vi "DHE_DO_IMREAD_NORMAL.vi"(8 "error in":errorcluster) -> (0 "error out":errorcluster, 2 "response":string)   [LabVIEW 2016]
uses:
  Common/public/vis/CMN_FVAR_action.ctl
  SDSU_GBLVariables.vi
  DBSHAND/private/vis/DatabaseHand_Element_Get(bool).vi
  DBSHAND/private/vis/DatabaseHand_Element_Get(double).vi
  DBSHAND/private/vis/DatabaseHand_Element_Set(double).vi
  c/lib/libarcDHE.so
panel:
  out "error out 2":errorcluster
  out "remaining elements":string[](array[string])
  in  "stop":bool
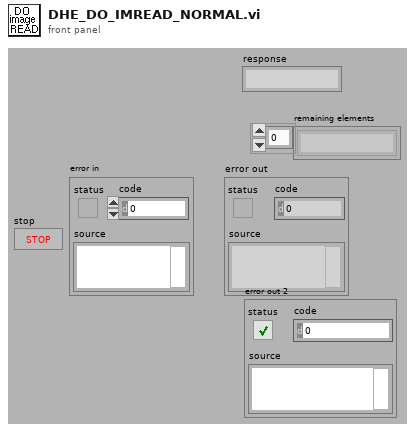
[diagram p1: front panel]
types:
  T1 = typedef "DatabaseHand_RefNum.ctl" = refnum<vi>
  T2 = enum16{"Idle", "Exposing", "Paused", "AbortExp", "Reading", "AbortRead", "FinishedReading", "Resetting", "Reducing"}
  T3 = cluster{"Video Processor Type":string, "support gain":bool, "Timing Board":string, "support reset":bool, "Utility Board":string, "Shutter":string, "Temperature":string, "support temp control":bool, "Detector Type":string, "Support MPP":string, "Support Binning":string, "Readout Mode":string, "support shutter control":bool}
  T4 = typedef "CMN_Buffers.ctl" = cluster{"TotalPixels":u32, "Total image bytes":u32, "Total Phys Buffers":u32, "virtual buf pixels":u32, "virtual bytes size":u32, "Remaining piece":u32, "Transfer_Buf_size":u32}
  T5 = typedef "CMN_TimingInfo.ctl" = cluster{"PixelTime":sgl, "SkipPixel":sgl, "SkipRow":sgl, "ShiftRow":sgl, "ShiftedPix":u16, "known_overhead":sgl, "DET_READ_TIME":sgl}
  T6 = typedef "CMN_FVAR_action.ctl" = enum16{"read", "write"}
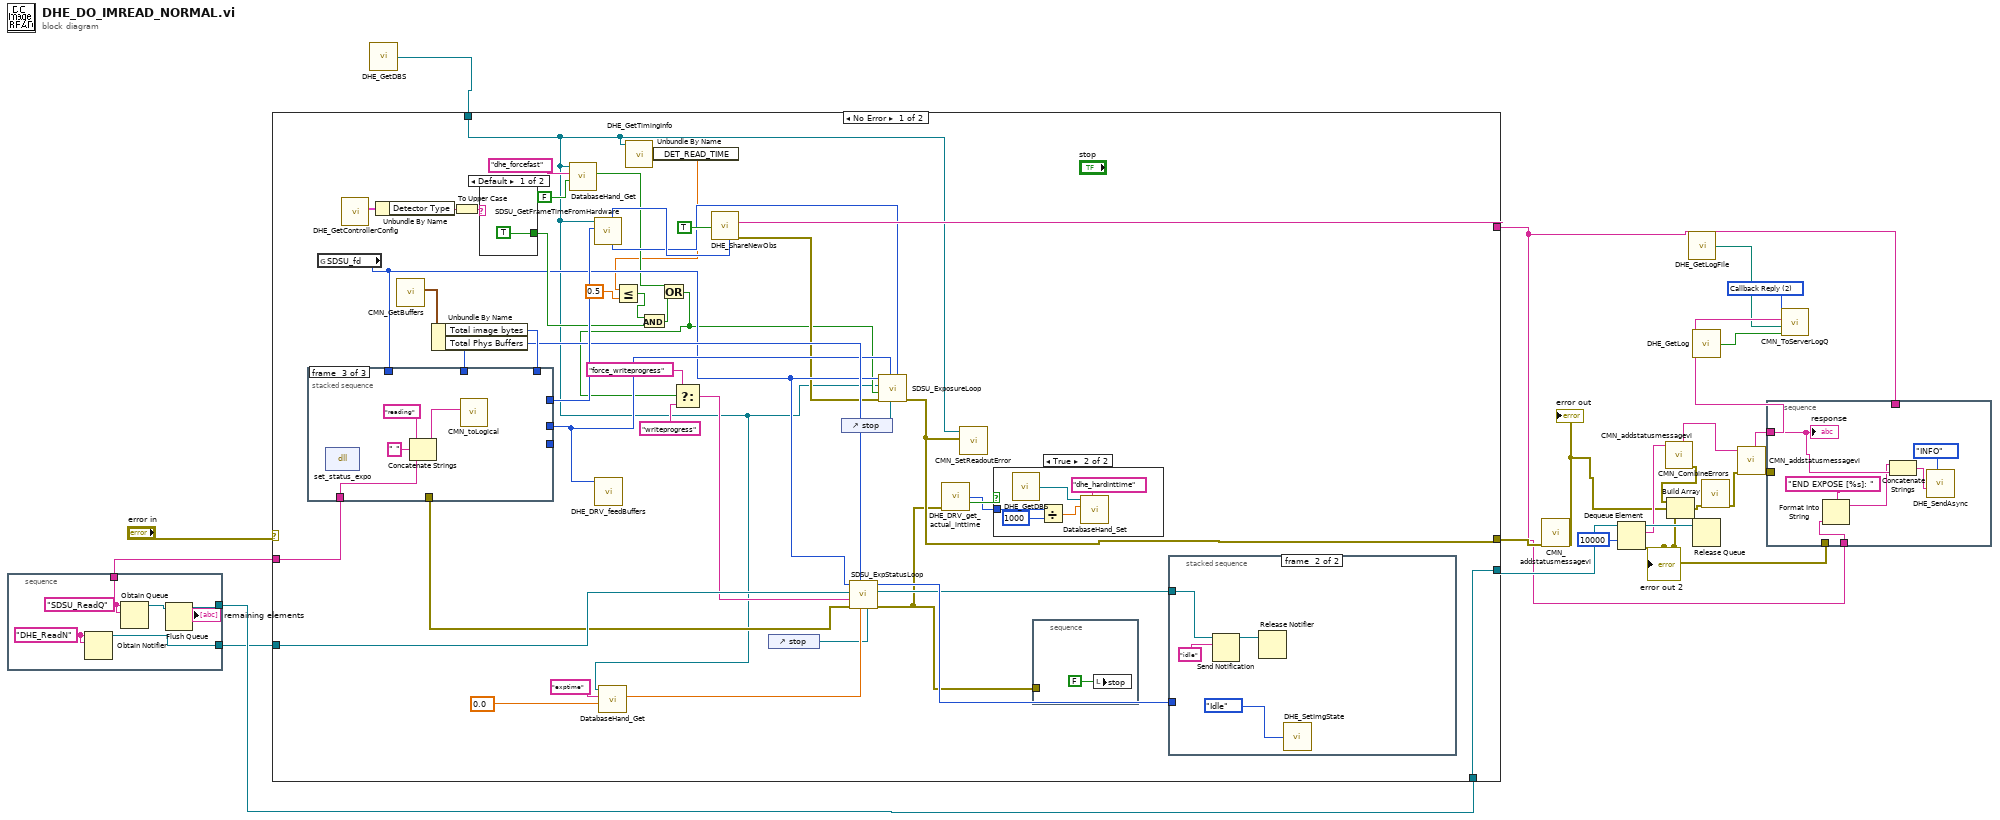
[diagram p0: block diagram]
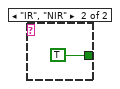
[diagram p3: hidden frame]
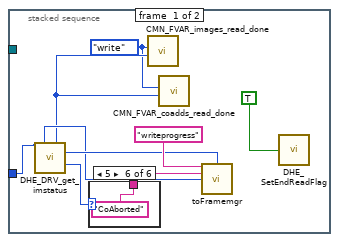
[diagram p4: hidden frame]
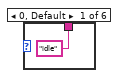
[diagram p5: hidden frame]
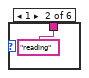
[diagram p6: hidden frame]
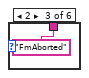
[diagram p7: hidden frame]
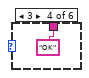
[diagram p8: hidden frame]
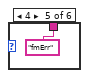
[diagram p9: hidden frame]
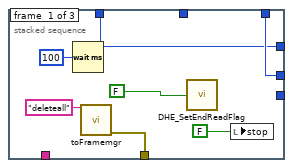
[diagram p10: hidden frame]
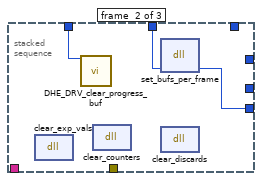
[diagram p11: hidden frame]
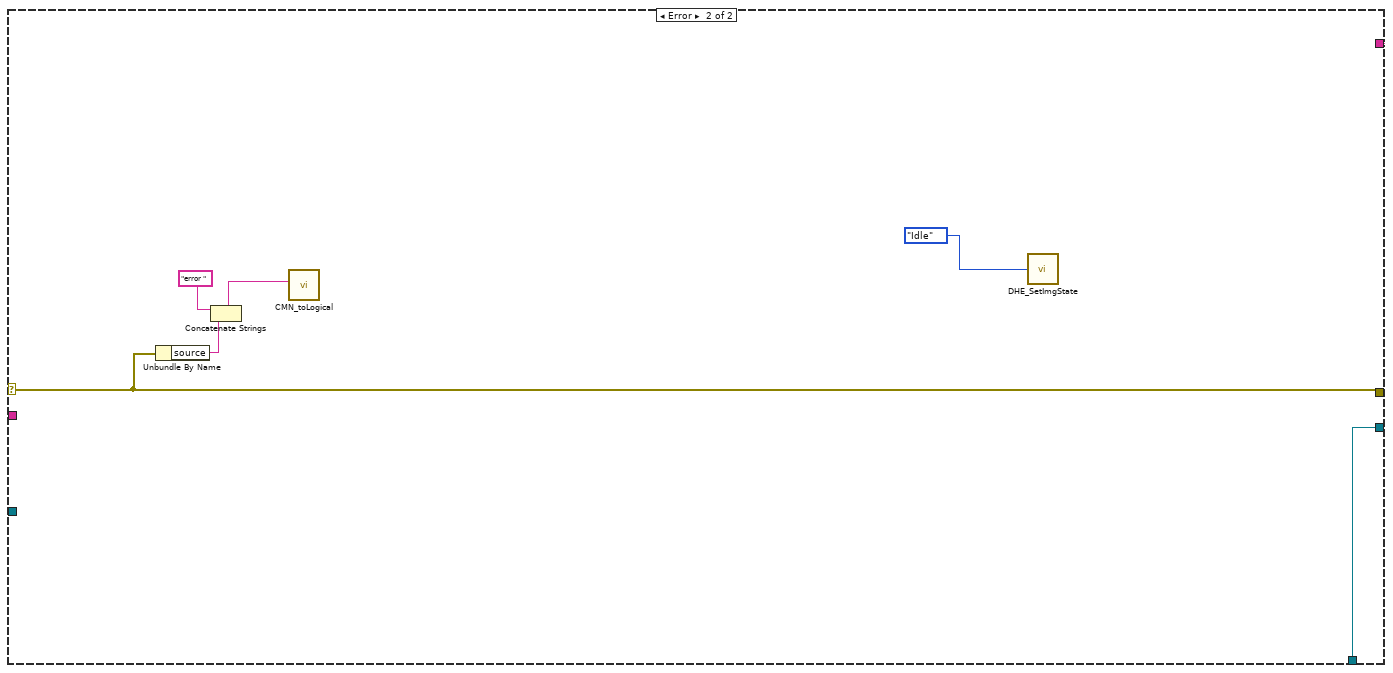
[diagram p12: hidden frame]
diagram:
  w19 = u16 2 items=["command", "imediateReply", "Callback Reply", "Information"] ("type")
  n1 = stacked-sequence {
    tunnel: [w28] -> w20
    tunnel: [w26] -> w15
    tunnel: [w23] -> w8
    frame #0 {
      w24 = "DHE_ReadN" ("name (unnamed)")
      w28 = "SDSU_ReadQ" ("name (unnamed)")
      n2 = Obtain Notifier(name (unnamed)=w24, notification data type=w24) -> (notifier out=w23:refnum<notifier>)  [unwired: 2 in, 2 out]
      n3 = Obtain Queue(name (unnamed)=w28, element data type=w28) -> (queue out=w27:refnum<queue>)  [unwired: 3 in, 2 out]
      n4 = Flush Queue(queue=w27) -> (queue out=w26:refnum<queue>, remaining elements=→"remaining elements":string[])  [unwired: 1 in, 1 out]
    }
  }
  n5 = call "DHE_GetDBS.vi"() -> ("DHE_DBSRef"=w5:T1)  [unwired: 9 out]
  n6 = case shown="No Error" "error in" {
    selector: "error in" -> [_ w118]
    tunnel: [w47 w118] -> w18
    tunnel: w5 -> [w34 _]
    tunnel: w20 -> [w68 _]
    tunnel: [w67 w115] -> w14
    tunnel: w15 -> [w67 w115]
    tunnel: w8 -> [w54 _]
    tunnel: [w62 "" ("obsID")] -> w2
    frame No Error {
      n7 = global read "SDSU_GBLVariables.vi" "SDSU_fd"() -> (w44:i32)
      n8 = call "DHE_GetControllerConfig.vi"() -> ("ControllerConfigCluster"=w58:T3)  [unwired: 11 out]
      n9 = Unbundle By Name(w58) -> ("Detector Type"=w57:string)
      n10 = call "CMN_GetBuffers.vi"() -> ("BuffersDimensions"=w69:T4)  [unwired: 2 in, 9 out]
      n11 = Unbundle By Name(w69) -> ("Total image bytes"=w66:u32, "Total Phys Buffers"=w52:u32)
      n12 = stacked-sequence {
        tunnel: [_ w106 _] -> _
        tunnel: w52 -> [_ w108 _]
        tunnel: w44 -> [w102 w107 _]
        tunnel: w68 -> [_ _ w110]
        tunnel: [w104 _ _] -> w45
        tunnel: w66 -> [w104 _ _]
        tunnel: [w102 _ _] -> w65
        tunnel: [w99 _ _] -> w48
        frame #0 {
          n13 = Wait (ms)(milliseconds to wait=u32 100) -> ()  [unwired: 1 out]
          n14 = call "toFramemgr.vi"("command"="deleteall") -> ("error out"=w99:errorcluster)  [unwired: 8 in, 6 out]
          n15 = call "DHE_SetEndReadFlag.vi"("DHE_read_ended"=FALSE ("readout ended")) -> ()  [unwired: 9 out]
          n16 = local write "stop"(FALSE ("stop")) -> ()
        }
        frame #1 {
          n17 = dll-call lib="home/simager/panview/PAN/Modules/SDSU/private/c/lib/libarcDHE.so" fn="clear_exp_vals"() -> ()  [unwired: 3 in, 3 out]
          n18 = call "DHE_DRV_clear_progress_buf.vi"("fd"=w107) -> ()  [unwired: 1 in, 14 out]
          n19 = dll-call lib="home/simager/panview/PAN/Modules/SDSU/private/c/lib/libarcDHE.so" fn="clear_counters"() -> ()  [unwired: 3 in, 3 out]
          n20 = dll-call lib="home/simager/panview/PAN/Modules/SDSU/private/c/lib/libarcDHE.so" fn="set_bufs_per_frame" label="bufs_per_frame"("total_bufs"=w108) -> ("total_bufs"=w106:i32)  [unwired: 3 in, 3 out]
          n21 = dll-call lib="home/simager/panview/PAN/Modules/SDSU/private/c/lib/libarcDHE.so" fn="clear_discards"() -> ()  [unwired: 3 in, 3 out]
        }
        frame #2 {
          n22 = dll-call lib="home/simager/panview/PAN/Modules/SDSU/private/c/lib/libarcDHE.so" fn="set_status_expo"() -> ()  [unwired: 3 in, 3 out]
          n23 = Concatenate Strings("reading" ("command"), " " ("string"), w110) -> (w109:string)
          n24 = call "CMN_toLogical.vi"("command"=w109) -> ()  [unwired: 10 out]
        }
      }
      n25 = To Upper Case(1:w57) -> (0:w56:string)
      n26 = case shown="Default" w56 {
        tunnel: [TRUE TRUE] -> w55
        frame Default {
        }
        frame "IR", "NIR" {
        }
      }
      n27 = call-poly "DatabaseHand_Get.vi"("default value"=FALSE ("async?"), "name"="dhe_forcefast", "Database RefNum in"=w34) -> ("value"=w36:bool)  [unwired: 2 in, 6 out]
      n28 = call "SDSU_GetFrameTimeFromHardware.vi"("fd"=w65, "Database Ref"=w34) -> ("idle time"=w43:u32, "total exp time"=w64:u32)  [unwired: 1 in, 7 out]
      n29 = call "DHE_DRV_feedBuffers.vi"("bufsize"=w45) -> ()  [unwired: 10 out]
      n30 = call-poly "DatabaseHand_Get.vi"("default value"=0.0, "name"="exptime", "Database RefNum in"=w34) -> ("value"=w51:dbl)  [unwired: 2 in, 6 out]
      n31 = call "DHE_GetTimingInfo.vi"("Database RefNum out"=w34) -> ("Timing"=w33:T5)  [unwired: 10 out]
      n32 = Unbundle By Name(w33) -> ("DET_READ_TIME"=w32:sgl)
      n33 = Less Or Equal?(x=w32, y=0.5) -> (x <= y?=w39:bool)
      n34 = And(x=w39, y=w55) -> (x .and. y?=w38:bool)
      n35 = Or(x=w36, y=w38) -> (x .or. y?=w37:bool)
      n36 = Select(t="force_writeprogress" ("command"), s=w37, f="writeprogress" ("command")) -> (s? t:f=w53:string)
      n37 = call "DHE_ShareNewObs.vi"("exptime (ms)"=w64, "async?"=TRUE) -> ("error out"=w42:errorcluster, "obsID"=w62:string)  [unwired: 1 in, 7 out]
      n38 = control-ref of="stop"() -> (w50:refnum<vi>)
      n39 = control-ref of="stop"() -> (w46:refnum<vi>)
      n40 = call "SDSU_ExpStatusLoop.vi"("stop ref"=w50, "exptime"=w51, "Total Phys Buffers"=w52, "error in (no error)"=w48, "frames command"=w53, "notifier"=w54, "fd"=w44) -> ("error out"=w29:errorcluster, "notifier  out"=w35:refnum<notifier>, "fd out"=w49:i32)  [unwired: 2 out]
      n41 = call "SDSU_ExposureLoop.vi"("idle time"=w43, "stop ref"=w46, "Total image bytes"=w45, "error IO"=w42, "fast"=w37, "Database RefNum in"=w34, "SDSU_fd"=w44) -> ("error out"=w47:errorcluster)  [unwired: 4 out]
      n42 = call "DHE_DRV_get_actual_inttime.vi"("error in (no error)"=w29) -> ("actual inttime"=w30:i32, "supported"=w31:bool)  [unwired: 13 out]
      n43 = call "CMN_SetReadoutError.vi"("readout error"=w47, "Database RefNum in"=w34) -> ()  [unwired: 1 in, 9 out]
      n44 = case shown="True" w31 {
        tunnel: w30 -> [_ w74]
        frame False {
        }
        frame True {
          n45 = call "DHE_GetDBS.vi"() -> ("DHE_DBSRef"=w76:T1)  [unwired: 9 out]
          n46 = Divide(x=w74, y=1000) -> (x/y=w72:dbl)
          n47 = call-poly "DatabaseHand_Set.vi"("name"="dhe_hardinttime", "value"=w72, "Database RefNum in"=w76) -> ()  [unwired: 5 in, 4 out]
        }
      }
      n48 = stacked-sequence {
        tunnel: w29 -> [_]
        frame #0 {
          n49 = local write "stop"(FALSE ("stop")) -> ()
        }
      }
      n50 = stacked-sequence {
        tunnel: w49 -> [w87 _]
        tunnel: w35 -> [_ w95]
        frame #0 {
          w80 = CMN_FVAR_action."write" ("action")
          n51 = call "DHE_DRV_get_imstatus.vi"("fd"=w87) -> ("ptr to buffer"=w83:u64, "buff read"=w84:i32, "frame status"=w86:i32, "images done"=w81:i32)  [unwired: 1 in, 10 out]
          n52 = case shown="5" w86 {
            tunnel: ["idle" "reading" "FmAborted" "OK" "fmErr" "CoAborted"] -> w85
            frame 0, Default {
            }
            frame 1 {
            }
            frame 2 {
            }
            frame 3 {
            }
            frame 4 {
            }
            frame 5 {
            }
          }
          n53 = call "CMN_FVAR_images_read_done.vi"("value in"=w81, "action"=w80) -> ()  [unwired: 9 out]
          n54 = call "CMN_FVAR_coadds_read_done.vi"("value in"=w81, "action"=w80) -> ()  [unwired: 9 out]
          n55 = call "toFramemgr.vi"("command"="writeprogress", "progress"=w84, "arg"=w85, "bufpointer"=w83) -> ()  [unwired: 5 in, 7 out]
          n56 = call "DHE_SetEndReadFlag.vi"("DHE_read_ended"=TRUE ("readout ended")) -> ()  [unwired: 9 out]
        }
        frame #1 {
          n57 = Send Notification(notification="idle", notifier=w95) -> (notifier out=w98:refnum<notifier>)  [unwired: 1 in, 1 out]
          n58 = Release Notifier(notifier=w98) -> ()  [unwired: 1 in, 4 out]
          n59 = call "DHE_SetImgState.vi"("DHE_ImgState"=T2."Idle" ("ImgState")) -> ()  [unwired: 9 out]
        }
      }
    }
    frame Error {
      n60 = Unbundle By Name(w118) -> ("source"=w117:string)
      n61 = Concatenate Strings("error " ("command"), w117) -> (w116:string)
      n62 = call "CMN_toLogical.vi"("command"=w116) -> ()  [unwired: 10 out]
      n63 = call "DHE_SetImgState.vi"("DHE_ImgState"=T2."Idle" ("ImgState")) -> ()  [unwired: 9 out]
    }
  }
  n64 = call "CMN_addstatusmessagevi.vi"("error in (no error)"=w18) -> ("error out"=w10:errorcluster)  [unwired: 1 in, 9 out]
  "error out" <- w10
  n65 = Dequeue Element(queue=w14, timeout in ms (-1)=10000) -> (queue out=w21:refnum<queue>, element=w12:string, error out=w3:errorcluster)  [unwired: 1 in, 1 out]
  "error out 2" <- w3
  n66 = call "CMN_addstatusmessagevi.vi"("message  in"=w12) -> ("error out"=w11:errorcluster, "modified message out"=w9:string)  [unwired: 1 in, 8 out]
  n67 = Build Array(w11, w10, w3) -> (w17:errorcluster[])
  n68 = call "DHE_GetLogFile.vi"() -> ("DHE_LogFile"=w6:path)  [unwired: 9 out]
  n69 = call "DHE_GetLog.vi"() -> ("DHE_log"=w7:bool)  [unwired: 9 out]
  n70 = Release Queue(queue=w21) -> ()  [unwired: 1 in, 4 out]
  n71 = call "CMN_CombineErrors.vi"("Errors"=w17) -> ("error out"=w16:errorcluster)  [unwired: 10 out]
  n72 = call "CMN_addstatusmessagevi.vi"("error in (no error)"=w16, "message  in"=w9) -> ("error out"=w4:errorcluster, "modified message out"=w13:string)  [unwired: 8 out]
  n73 = stacked-sequence {
    tunnel: w13 -> [w124]
    tunnel: w4 -> [_]
    tunnel: w3 -> [_]
    tunnel: w2 -> [_]
    tunnel: w2 -> [w122]
    frame #0 {
      n74 = Format Into String(format string="END EXPOSE [%s]: " ("string"), w122) -> (resulting string=w121:string)  [unwired: 2 in, 1 out]
      n75 = Concatenate Strings(w121, w124) -> (w120:string)
      n76 = call "DHE_SendAsync.vi"("type"=enum16{"ERROR", "WARNING", "INFO", "CHANGED"}."INFO", "Message"=w120) -> ()  [unwired: 2 in, 8 out]
      "response" <- w124
    }
  }
  n77 = call "CMN_ToServerLogQ.vi"("Log"=w7, "file"=w6, "string"=w13, "type"=w19) -> ()  [unwired: 2 in, 5 out]
